vi "Open.vi"(8 "error in (no error)":errorcluster, 9 "Operation":T1, 10 "Path":path, 11 "Data.TDMS in":refnum<class "LV-Data.TDMS.lvclass">) -> (0 "error out":errorcluster, 3 "Data.TDMS out":refnum<class "LV-Data.TDMS.lvclass">)   [LabVIEW 2016, in "LV-Data.TDMS.lvclass"]
uses:
  LV-Data.TDMS.lvclass
  C:/Users/patrick/Documents/GitHub/LV-to-ITX/src/LV-Data/LV-Data.lvclass
  LV-Data/Typedefs/Operation--enum.ctl
  LV-Data/LV-Data.lvclass/LV-Data.ctl
  LV-Data.TDMS.lvclass/LV-Data.TDMS.ctl
  LV-Data/LV-Data.lvclass
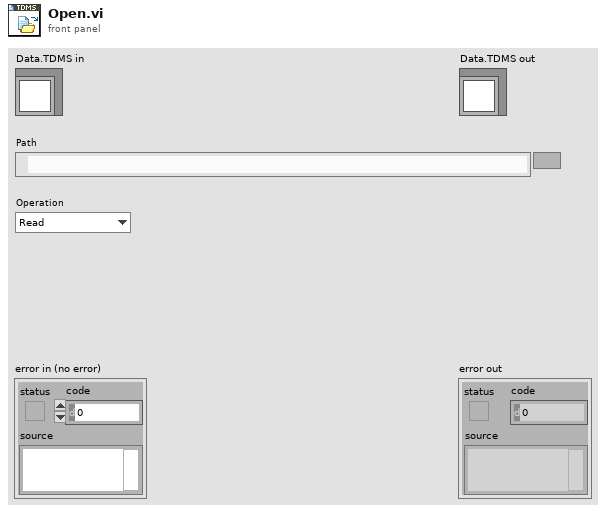
[diagram p1: front panel]
types:
  T1 = typedef "LV-Data.lvclass/Operation--enum.ctl" = enum16{"Read", "Write", "Write + Append"}
  T2 = enum16{"open", "open or create", "create or replace", "create", "open (read-only)"}
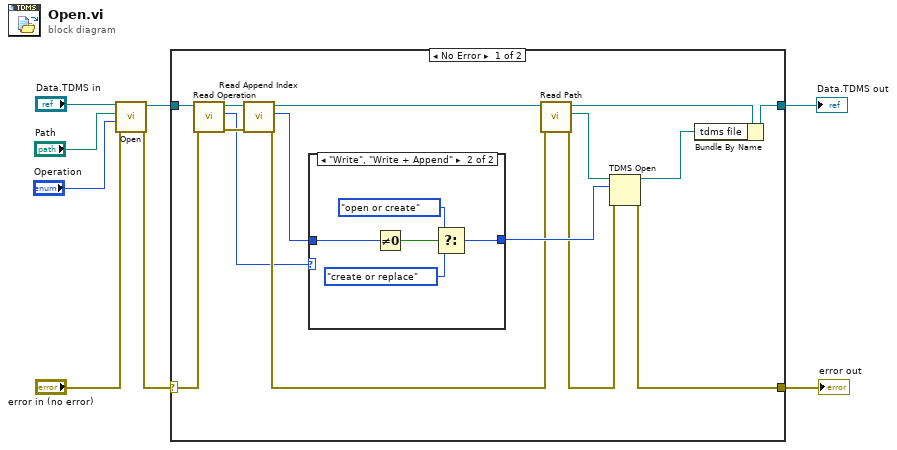
[diagram p0: block diagram]
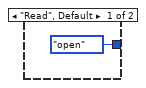
[diagram p2: hidden frame]
diagram:
  n1 = call-parent "Open.vi"("error in (no error)"="error in (no error)", "Operation"="Operation", "Path"="Path", "Data in"="Data.TDMS in") -> ("error out"=w6:errorcluster, "Data out"=w4:refnum<class "LV-Data.TDMS.lvclass">)  [unwired: 6 in]
  n2 = case shown="No Error" w6 {
    selector: w6 -> [w11 w31]
    tunnel: [w22 w31] -> w5
    tunnel: w4 -> [w13 w30]
    tunnel: [w17 w30] -> w3
    frame No Error {
      n3 = call "Read Operation.vi"("error in (no error)"=w11, "Data in"=w13) -> ("error out"=w10:errorcluster, "Operation"=w9:T1, "Data out"=w12:refnum<class "LV-Data.TDMS.lvclass">)  [unwired: 7 in]
      n4 = call "Read Append Index.vi"("error in (no error)"=w10, "Data in"=w12) -> ("error out"=w15:errorcluster, "Append Index"=w14:i32, "Data out"=w16:refnum<class "LV-Data.TDMS.lvclass">)  [unwired: 7 in]
      n5 = case shown="\"Write\", \"Write + Append\"" w9 {
        tunnel: [T2."open" ("operation (0:open)") w29] -> w23
        tunnel: w14 -> [_ w26]
        frame "Read", Default {
        }
        frame "Write", "Write + Append" {
          n6 = Not Equal To 0?(x=w26) -> (x != 0?=w25:bool)
          n7 = Select(t=T2."open or create" ("operation (0:open)"), s=w25, f=T2."create or replace" ("operation (0:open)")) -> (s? t:f=w29:T2)
        }
      }
      n8 = call "Read Path.vi"("error in (no error)"=w15, "Data Save"=w16) -> ("error out"=w20:errorcluster, "Path"=w21:path, "Data Save out"=w19:refnum<class "LV-Data.TDMS.lvclass">)  [unwired: 7 in]
      n9 = TDMS Open(8:w20, 10:w23, 11:w21) -> (0:w22:errorcluster, 3:w18:refnum<k34>)  [unwired: 4 in]
      n10 = Bundle By Name(cluster=w19, "tdms file"=w18) -> (w17:refnum<class "LV-Data.TDMS.lvclass">)
    }
    frame Error {
    }
  }
  "error out" <- w5
  "Data.TDMS out" <- w3
